vi "Calculate tds Factor.vi"(8 "error in (no error)":errorcluster, 9 "tds Value":dbl, 10 "Channel":T1, 11 "EPU452 in":refnum<class "EPU452.lvclass">) -> (0 "error out":errorcluster, 1 "tds Factor":dbl, 2 "Response":string, 3 "EPU452 out":refnum<class "EPU452.lvclass">)   [LabVIEW 2018, in "EPU452.lvclass"]
uses:
  EPU452.lvclass
  Controls/Channels.ctl
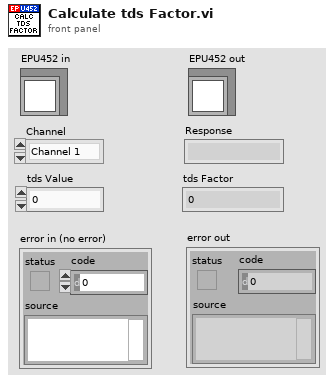
[diagram p1: front panel]
types:
  T1 = typedef "EPU452.lvclass/Channels.ctl" = enum16{"Channel 1", "Channel 2", "Channel 3", "Channel 4"}
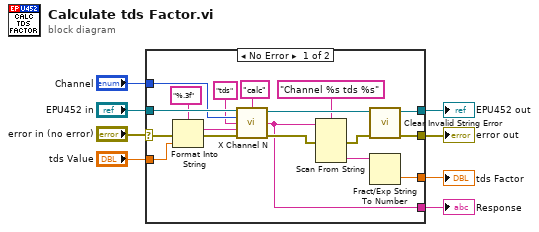
[diagram p0: block diagram]
diagram:
  n1 = case shown="No Error" "error in (no error)" {
    selector: "error in (no error)" -> [w23 w28]
    tunnel: [w16 w28] -> w7
    tunnel: [w17 w27] -> w5
    tunnel: "EPU452 in" -> [w26 w27]
    tunnel: "Channel" -> [w25 _]
    tunnel: "tds Value" -> [w20 _]
    tunnel: [w9 _] -> w2
    tunnel: [w10 _] -> w1
    frame No Error {
      n2 = Format Into String(format string="%.3f", error in=w23, w20) -> (resulting string=w21:string, error out=w22:errorcluster)  [unwired: 1 in]
      n3 = call "X Channel N.vi"("EPU452 in"=w26, "Operation"="calc", "Channel"=w25, "Function"="tds", "Argument/s"=w21, "error in (no error)"=w22) -> ("EPU452 out"=w15:refnum<class "EPU452.lvclass">, "Response"=w9:string, "error out"=w13:errorcluster)  [unwired: 7 in]
      n4 = Scan From String(format string="Channel %s tds %s", input string=w9, error in=w13) -> (error out=w14:errorcluster, output 2=w11:string)  [unwired: 4 in, 2 out]
      n5 = call "Clear Invalid String Error.vi"("error in (no error)"=w14, "EPU452 in"=w15) -> ("error out"=w16:errorcluster, "EPU452 out"=w17:refnum<class "EPU452.lvclass">)  [unwired: 8 in]
      n6 = Fract/Exp String To Number(string=w11) -> (number=w10:dbl)  [unwired: 3 in, 1 out]
    }
    frame Error {
    }
  }
  "error out" <- w7
  "EPU452 out" <- w5
  "Response" <- w2
  "tds Factor" <- w1
